vi "draw_track6_close&dis&angle_resist.vi"(2 "GOALpos":cluster{"X":sgl, "Y":sgl}[](array[cluster]), 3 "角度阈值":dbl=60.0 format="%#_13g", 4 "距离阈值":dbl=1000.0 format="%#_13g", 5 "bin_billard":T1, 6 "color_billard":T1) -> (0 "new picture":picture caption="新图片", 1 "大小":i32)   [LabVIEW 2018]
uses:
  <vilib>/vision/Shape Detection.llb/ShapeDetectionMatchOptions.ctl
  <vilib>/vision/Pattern Matching.llb/IMAQ Match Range Setting.ctl
  <vilib>/vision/Image Controls.llb/IMAQ Image.ctl
  <vilib>/vision/NI_Vision_Development_Module.lvlib
panel:
  in  "Match Options":T2 {"Range Settings"."Match Constraints" items=["Rotation Angle (degrees)", "Scale Factor (%)", "Occlusion (%)"]}
  out "endX":dbl format="%#_13g"
  out "endY":dbl format="%#_13g"
  # "Range"
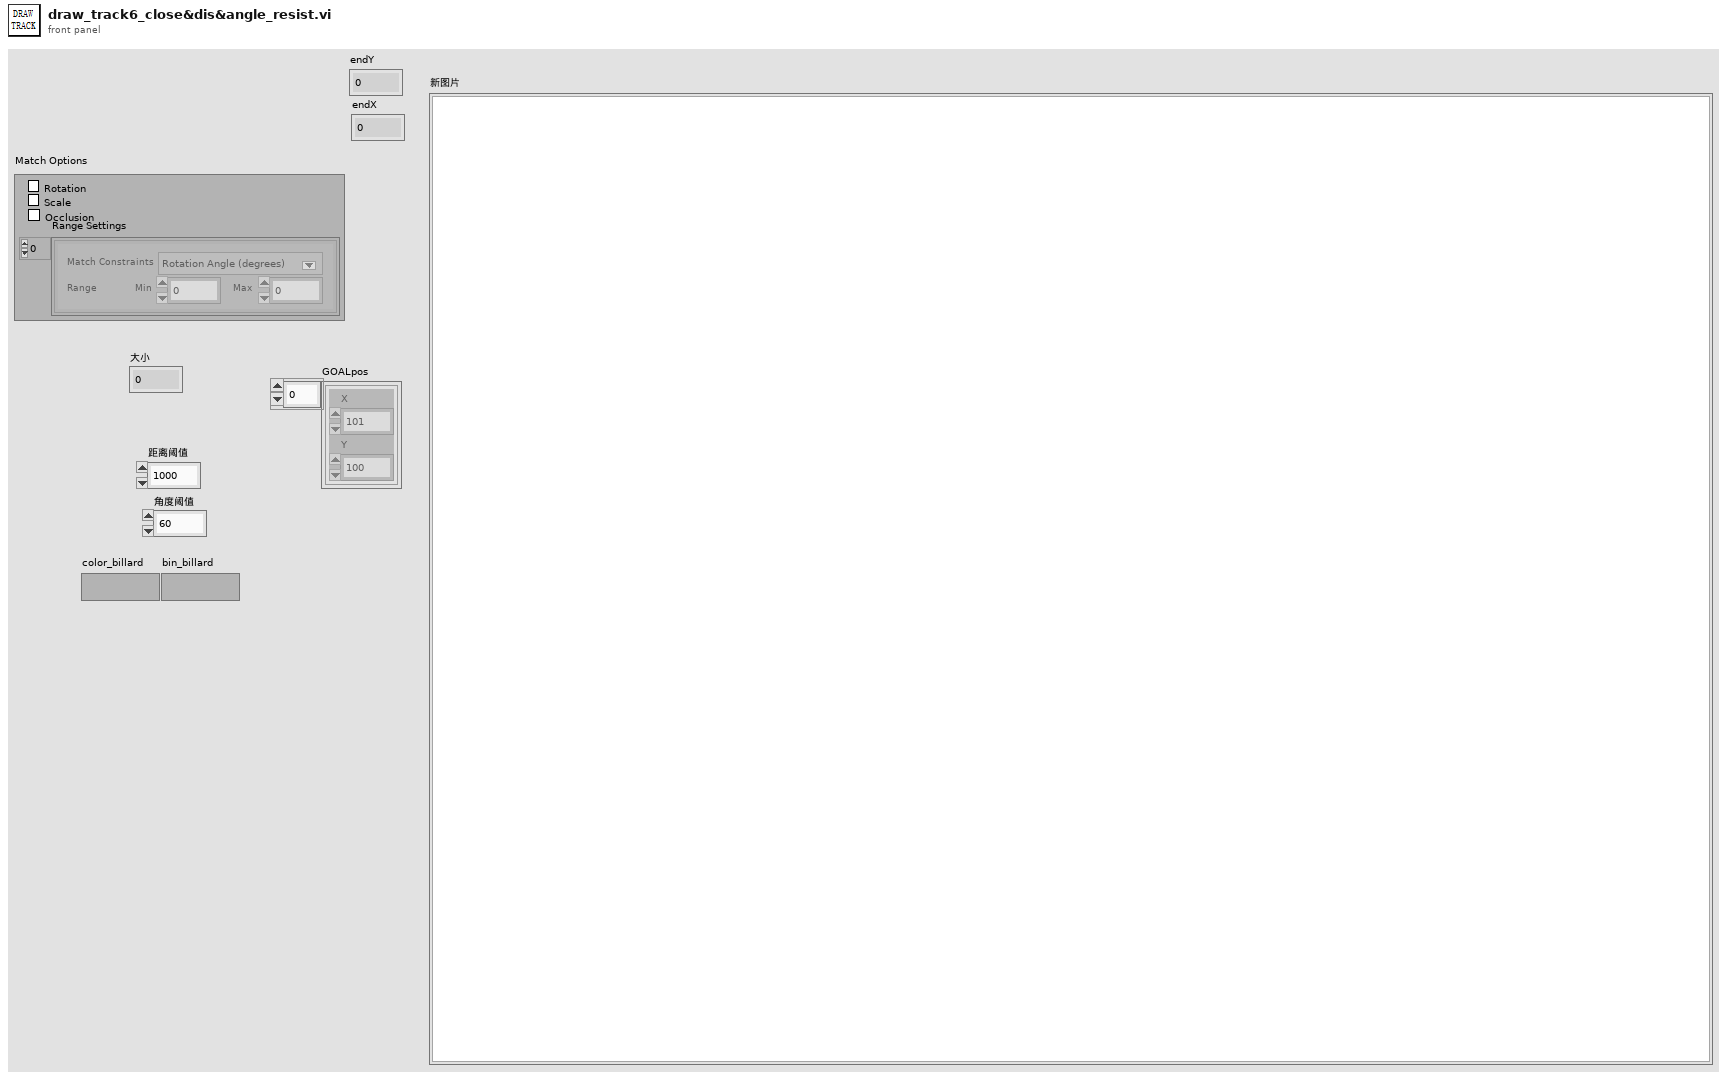
[diagram p1: front panel]
types:
  T1 = typedef "IMAQ Image.ctl" = refnum<image>
  T2 = typedef "ShapeDetectionMatchOptions.ctl" = cluster{"Rotation":bool, "Scale":bool, "Occlusion":bool, "Range Settings":T3[]}
  T3 = typedef "IMAQ Match Range Setting.ctl" = cluster{"Match Constraints":u32, "Min":dbl, "Max":dbl}
  T4 = cluster{"Position":cluster{"X":sgl, "Y":sgl}, "Radius":dbl, "Score":dbl}[]
  T5 = cluster{"Position":cluster{"X":sgl, "Y":sgl}, "Radius":dbl, "Score":dbl}
  T6 = cluster{i32, i32, "X Resolution":i32, "Y Resolution":i32}
  T7 = cluster{"Width":u16, "Style":enum32{"Solid", "Dash", "Dot", "DashDot", "DashDotDot"}}
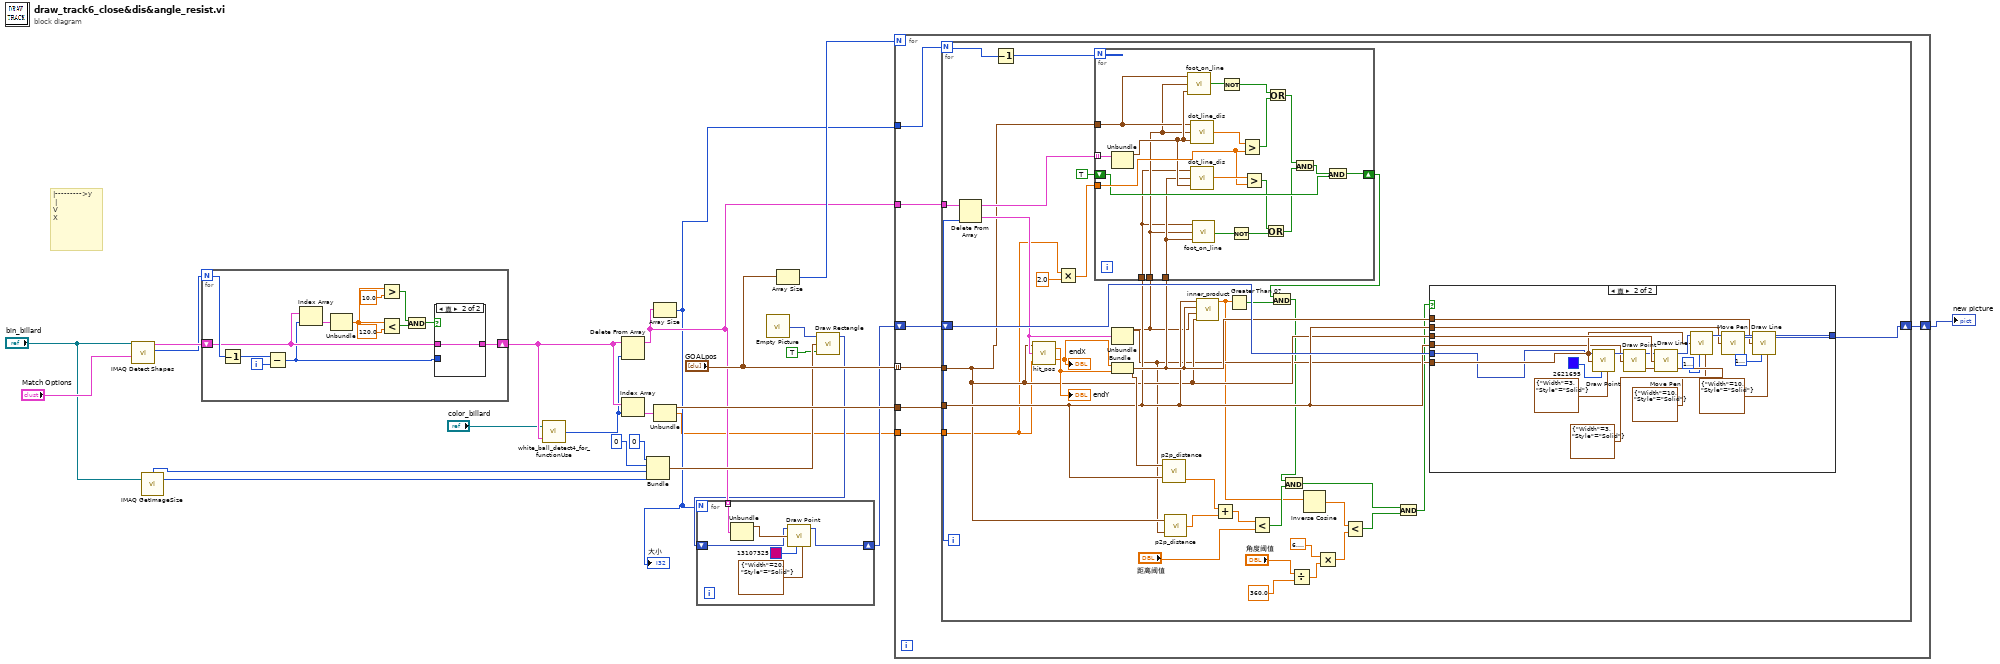
[diagram p0: block diagram]
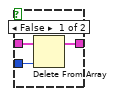
[diagram p3: hidden frame]
diagram:
  # "|--------->y\n |\nV\nX"
  n1 = call-poly "IMAQ Detect Shapes"("Match Options"="Match Options", "Image"="bin_billard") -> ("Number of Matches Returned"=w22:i32, "Circles"=w23:T4)  [unwired: 7 in, 1 out]
  n2 = call "IMAQ GetImageSize"("Image"="bin_billard") -> ("Y Resolution"=w9:i32, "X Resolution"=w8:i32)  [unwired: 3 in, 1 out]
  n3 = for {
    N: w22 -> [w32]
    shift-right: [w26] -> w16
    shift-left: w23 -> [w27]
    i -> [w30]
    n4 = Decrement(x=w32) -> (x-1=w31:i32)
    n5 = Subtract(x=w31, y=w30) -> (x-y=w25:i32)
    n6 = Index Array(array=w27, index=w25) -> (element=w29:T5)
    n7 = Unbundle(w29) -> ("Radius"=w36:dbl)  [unwired: 2 out]
    n8 = Greater?(x=w36, y=10.0) -> (0:w34:bool)
    n9 = Less?(x=w36, y=120.0) -> (x < y?=w33:bool)
    n10 = And(x=w34, y=w33) -> (x .and. y?=w28:bool)
    n11 = case shown="真" w28 {
      tunnel: w27 -> [w40 w41]
      tunnel: [w39 w41] -> w26
      tunnel: w25 -> [w38 _]
      frame False {
        n12 = Delete From Array(array=w40, index=w38) -> (array with subset deleted=w39:T4)  [unwired: 1 in, 1 out]
      }
      frame True {
      }
    }
  }
  n13 = call "white_ball_detect4_for_functionUse.vi"("Circles"=w16, "color_billard"="color_billard") -> ("白球所在(已处理的)数组位置"=w14:i32)
  n14 = Delete From Array(array=w16, index=w14) -> (array with subset deleted=w5:T4)  [unwired: 1 in, 1 out]
  n15 = Index Array(array=w16, index=w14) -> (element=w21:T5)
  n16 = Bundle(0, 0, "X Resolution"=w8, "Y Resolution"=w9) -> (w7:T6)  [unwired: 1 in]
  n17 = Array Size(array=w5) -> (size(s)=w2:i32)
  "大小" <- w2
  n18 = Unbundle(w21) -> ("Position"=w20:cluster{"X":sgl, "Y":sgl}, "Radius"=w1:dbl)  [unwired: 1 out]
  n19 = call "Empty Picture"() -> ("empty picture"=w12:picture)
  n20 = Array Size(array="GOALpos") -> (size(s)=w17:i32)
  n21 = call <vilib>:"Draw Rectangle.vi"("picture"=w12, "rect"=w7, "fill?(F)"=TRUE) -> ("new picture"=w4:picture)  [unwired: 6 in]
  n22 = for {
    N: w2 -> [_]
    tunnel: w5 -> [w47] mode=indexing
    shift-right: [w44] -> w3
    shift-left: w4 -> [w45]
    n23 = Unbundle(w47) -> ("Position"=w46:cluster{"X":sgl, "Y":sgl})  [unwired: 2 out]
    n24 = call <vilib>:"Draw Point.vi"("picture"=w45, "point(x,y)"=w46, "color(black)"=u32 13107325, "pen"=T7 {"Width"=20, "Style"=enum."Solid"}) -> ("new picture"=w44:picture)  [unwired: 5 in]
  }
  n25 = for {
    N: w17 -> [_]
    tunnel: w20 -> [w54]
    tunnel: w2 -> [w53]
    tunnel: "GOALpos" -> [w52] mode=indexing
    tunnel: w5 -> [w49]
    shift-right: [w50] -> w19
    shift-left: w3 -> [w51]
    tunnel: w1 -> [w48]
    n26 = for {
      N: w53 -> [w86]
      tunnel: w54 -> [w76]
      tunnel: w52 -> [w75]
      shift-right: [w89] -> w50
      shift-left: w51 -> [w90]
      tunnel: w49 -> [w80]
      tunnel: w48 -> [w56]
      i -> [w81]
      n27 = Delete From Array(array=w80, index=w81) -> (deleted portion=w79:T5, array with subset deleted=w84:T4)  [unwired: 1 in]
      n28 = Decrement(x=w86) -> (x-1=w85:i32)
      n29 = call "hit_pos.vi"("radius"=w56, "TARGET Circle Descriptor"=w79, "GOALpos"=w75) -> ("endX"=w87:dbl, "endY"=w88:dbl)
      "endY" <- w88
      "endX" <- w87
      n30 = Multiply(x=w56, y=2.0) -> (x*y=w55:dbl)
      n31 = Unbundle(w79) -> ("Position"=w74:cluster{"X":sgl, "Y":sgl})  [unwired: 2 out]
      n32 = Bundle("endX"=w87, "endY"=w88) -> (w77:cluster{"endX":dbl, "endY":dbl})  [unwired: 1 in]
      n33 = for {
        N: w85 -> [_]
        tunnel: w75 -> [w94]
        tunnel: w84 -> [w110] mode=indexing
        tunnel: w74 -> [w92]
        tunnel: w76 -> [w91]
        tunnel: w77 -> [w93]
        tunnel: w55 -> [w107]
        shift-right: [w104] -> w78
        shift-left: TRUE -> [w105]
        n34 = Unbundle(w110) -> ("Position"=w95:cluster{"X":sgl, "Y":sgl})  [unwired: 2 out]
        n35 = call "foot_on_line.vi"("dot"=w95, "line end"=w92, "line start"=w94) -> ("foot on line？"=w102:bool)
        n36 = call "dot_line_dis.vi"("dot pos"=w95, "line end"=w92, "line start"=w94) -> ("distance"=w109:sgl)
        n37 = call "dot_line_dis.vi"("dot pos"=w95, "line end"=w93, "line start"=w91) -> ("distance"=w108:sgl)
        n38 = call "foot_on_line.vi"("dot"=w93, "line end"=w92, "line start"=w91) -> ("foot on line？"=w103:bool)
        n39 = Not(x=w102) -> (.not. x?=w100:bool)
        n40 = Not(x=w103) -> (.not. x?=w101:bool)
        n41 = Greater?(x=w109, y=w107) -> (0:w99:bool)
        n42 = Greater?(x=w108, y=w107) -> (0:w98:bool)
        n43 = Or(x=w98, y=w101) -> (x .or. y?=w96:bool)
        n44 = Or(x=w100, y=w99) -> (x .or. y?=w97:bool)
        n45 = And(x=w97, y=w96) -> (x .and. y?=w106:bool)
        n46 = And(x=w106, y=w105) -> (x .and. y?=w104:bool)
      }
      n47 = call "p2p_distance.vi"("point2"=w76, "point1"=w77) -> ("poit2poit_dis"=w73:dbl)
      n48 = call "p2p_distance.vi"("point2"=w74, "point1"=w75) -> ("poit2poit_dis"=w72:dbl)
      n49 = call "inner_product.vi"("L2ENDpos"=w75, "L2STARTpos"=w74, "L1ENDpos"=w77, "L1STARTpos"=w76) -> ("数值"=w67:dbl)  [unwired: 7 in]
      n50 = Add(x=w73, y=w72) -> (x+y=w71:dbl)
      n51 = Greater Than 0?(x=w67) -> (x > 0?=w83:bool)
      n52 = Less?(x=w71, y="距离阈值") -> (x < y?=w68:bool)
      n53 = And(x=w78, y=w83) -> (x .and. y?=w69:bool)
      n54 = And(x=w69, y=w68) -> (x .and. y?=w64:bool)
      n55 = Divide(x="角度阈值", y=360.0) -> (x/y=w60:dbl)
      n56 = Inverse Cosine(1:w67) -> (0:w66:dbl)
      n57 = Multiply(x=6.283185307179586, y=w60) -> (x*y=w61:dbl)
      n58 = Less?(x=w66, y=w61) -> (x < y?=w65:bool)
      n59 = And(x=w64, y=w65) -> (x .and. y?=w63:bool)
      n60 = case shown="真" w63 {
        tunnel: w75 -> [_ w124]
        tunnel: w90 -> [w111 w112]
        tunnel: w74 -> [_ w122]
        tunnel: w76 -> [_ w129]
        tunnel: w77 -> [_ w127]
        tunnel: [w111 w126] -> w89
        tunnel: w76 -> [_ w118]
        frame False {
        }
        frame True {
          n61 = call <vilib>:"Draw Point.vi"("picture"=w112, "point(x,y)"=w122, "color(black)"=u32 2621695, "pen"=T7 {"Width"=3, "Style"=enum."Solid"}) -> ("new picture"=w120:picture)  [unwired: 5 in]
          n62 = call <vilib>:"Draw Point.vi"("picture"=w120, "point(x,y)"=w118, "pen"=T7 {"Width"=3, "Style"=enum."Solid"}) -> ("new picture"=w119:picture)  [unwired: 6 in]
          n63 = call <vilib>:"Move Pen.vi"("new position"=w124, "picture"=w119) -> ("new picture"=w125:picture)  [unwired: 3 in]
          n64 = call <vilib>:"Draw Line.vi"("picture"=w125, "end point"=w122, "color(black)"=u32 16777226, "pen"=T7 {"Width"=10, "Style"=enum."Solid"}) -> ("new picture"=w130:picture)  [unwired: 5 in]
          n65 = call <vilib>:"Move Pen.vi"("new position"=w129, "picture"=w130) -> ("new picture"=w128:picture)  [unwired: 3 in]
          n66 = call <vilib>:"Draw Line.vi"("picture"=w128, "end point"=w127, "color(black)"=u32 16777226, "pen"=T7 {"Width"=10, "Style"=enum."Solid"}) -> ("new picture"=w126:picture)  [unwired: 5 in]
        }
      }
    }
  }
  "new picture" <- w19
